vi "Camera.v6.vi"() -> ()   [LabVIEW 2015]
uses:
  Camera Properties.ctl
  Microscope Settings.ctl
  CameraState.ctl
  ModeEnum.ctl
  Stack_State.ctl
  Stack Track.ctl
  CameraControlTypeDef.ctl
  <vilib>/DAQmx/write.llb/DAQmx Write (Digital 1D Wfm NChan NSamp).vi
  <vilib>/DAQmx/write.llb/DAQmx Write (Analog 1D Wfm NChan NSamp).vi
  <vilib>/DAQmx/create/channels.llb/DAQmx Create Channel (AO-Voltage-Basic).vi
  <vilib>/Waveform/WDTOps.llb/WDT Number of Waveform Samples DBL.vi
  <vilib>/DAQmx/configure/timing.llb/DAQmx Timing (Sample Clock).vi
  <vilib>/Waveform/DWDTOps.llb/DWDT Uncompress Digital.vi
  <vilib>/DAQmx/miscellaneous.llb/DAQmx Fill In Error Info.vi
  <vilib>/vision/NI_Vision_Development_Module.lvlib
panel:
  in  "Tab Control":enum32{"Camera Settings", "Recording"}(tab)
  in  "Microscope Settings":T1={"Mode"=enum."XY", {"Scanning Mode"=12.0, "Slit Width /%"=5.0}, "Piezo Position /um"=0.0, "Exposure/ms"=40.0, "Samples per millisecond"=100.0, "Relax/ms"=10.0, "Readout Direction"=2.0, "Trigger Source"=2.0} {"Trigger Source" items=["Internal"=1.0, "External"=2.0]; "Readout Direction" items=["Forward"=1.0, "Backward"=2.0]; "?"."Scanning Mode" items=["Full Frame"=1.0, "Slit Scanning"=12.0]}
  in  "Scan":bool
  in  "Scan Continuously":bool
  out "error IO":errorcluster
  in  "V Height":dbl=2048.0 min=4.0 max=2048.0 step=4.0
  in  "V Offset":dbl min=0.0 max=0.0 step=4.0
  in  "H Offset":dbl min=0.0 max=0.0 step=4.0
  in  "H Width":dbl min=4.0 max=2048.0 step=4.0
  in  "Advanced DCAM Controls":i32(listbox) caption="Multicolumn Listbox"
  in  "Properties":T2=4211904 items=["SENSOR MODE"=4212128, "CCD MODE"=4212384, "READOUT MODE"=4211872, "ACTIVE VIEW INDEX"=4343136, "BITS PER CHANNEL"=4342976, "IMAGE PIXEL TYPE"=4343296, "BINNING"=4215968, "EXPOSURE TIME"=2049184, "CONTRAST GAIN"=3163312, "CONTRAST OFFSET"=3163328, "LIGHT MODE"=2114720, "SENSITIVITY"=2114992, "PHOTON IMAGING MODE"=2115200, "HIGH DYNAMIC RANGE MODE"=3163360, "WHITE BALANCE"=3163568, "TEMPERATURE"=2115232, "TEMPERATURE TARGET"=2115264, "SENSOR COOLER FAN"=2115296, "LINEBUNDLE HEIGHT"=4212192, "MECHANICAL SHUTTER"=2115488, "BACK FOCUS POSITION"=8422304, "TRIGGER CONNECTOR"=1066432, "TRIGGER SOURCE"=1066144, "OUTPUT TRIGGER SOURCE"=1852576, "TRIGGER GLOBAL EXPOSURE"=2049680, "FIRST TRIGGER BEHAVIOR"=2049696, "CHANNEL SYNC"=1852352, "READOUT DIRECTION"=4211904, "PRE HSYNC COUNT"=1852704, "INTERNAL LINE SPEED"=4191408, "INTERNAL LINE INVERVAL"=4191424]
  out "Waves":waveform(dbl)[](graph)
  out "Image":T3(plugin-control)
  out "Histogram":T4(graph)
  in  "stop":bool
  in  "Calibration":bool
  in  "MultiD Scan":bool
  in  "Stage Controller":bool
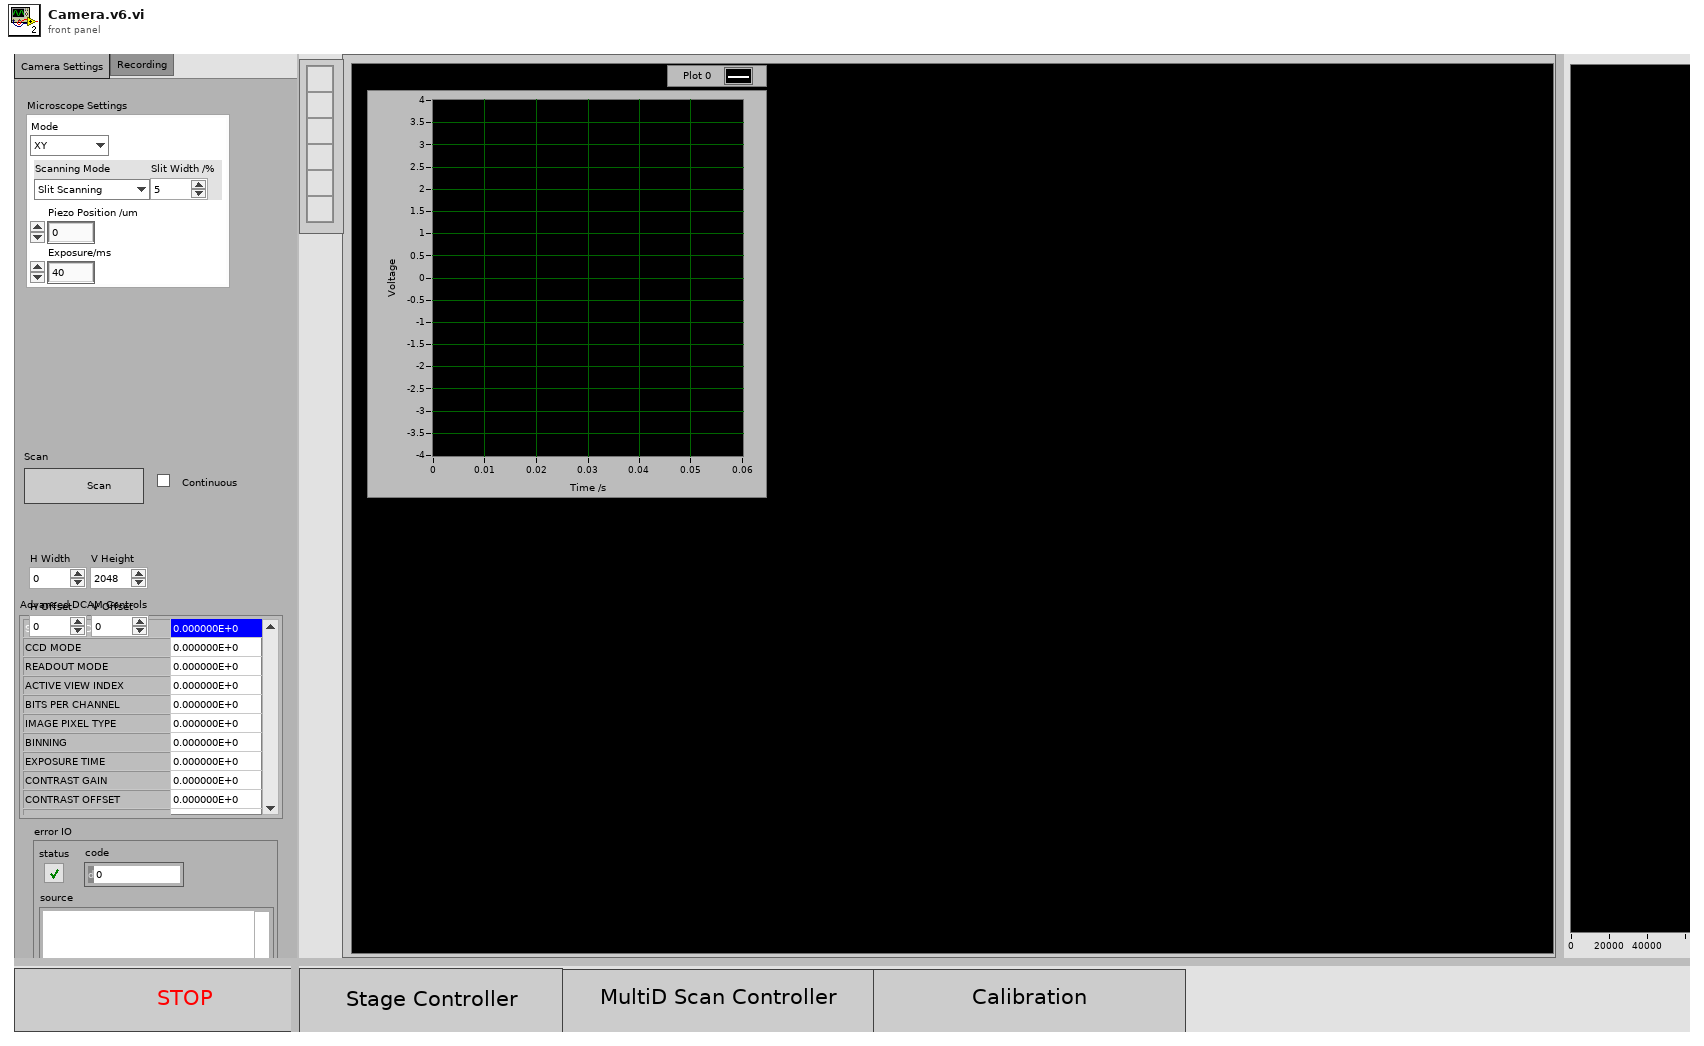
[diagram p1: front panel]
types:
  T1 = typedef "Microscope Settings.ctl" = cluster{"Mode":enum16{"X", "XY", "XYZ", "XYZT", "XYZC"}, cluster{"Scanning Mode":dbl, "Slit Width /%":dbl}, "Piezo Position /um":dbl, "Exposure/ms":dbl, "Samples per millisecond":dbl, "Relax/ms":dbl, "Readout Direction":dbl, "Trigger Source":dbl}
  T2 = typedef "Camera Properties.ctl" = u32
  T3 = typedef "IMAQ Image.ctl" = refnum<image>
  T4 = cluster{"Starting Value":sgl, "Incremental Value":sgl, "Histogram":u32[]}
  T5 = cluster{"height":u32, "width":u32, "datatype":u32}
  T6 = typedef "CameraState.ctl" = enum16{"init", "active", "deinit"}
  T7 = typedef "ModeEnum.ctl" = enum16{"Idle", "generateWaves", "runWaves", "stop"}
  T8 = typedef "CameraControlTypeDef.ctl" = enum16{"IntervalLineInt", "Ram Record", "HardDisk Record", "Disengage Update", "Update", "Idle", "ROI", "Binning", "Scan Mode", "Trigger Mode", "Readout Mode", "Readout Direction", "Preview", "ROIWindow", "Trigger Source"}
  T9 = typedef "Stack_State.ctl" = cluster{"State":T10, "Stack Number":i32, "Image":u16[][], "Stacks":i32}
  T10 = typedef "Stack Track.ctl" = enum16{"Idle", "Display", "Start Sequence", "Read Disk", "STOP", "Collecting", "End"}
  T11 = typedef "Image Type" = u32
  T12 = cluster{"Value":i32, "Minimum":i32, "Maximum":i32, "Increment":i32}
  T13 = cluster{"Minimum":i32, "Maximum":i32, "Increment":i32}
  T14 = cluster{"State":T10, "Timeout":i32, "Data 16":u16[][], "Timeout":i32}
  T15 = cluster{"Enum":T8, "Trigger Source":dbl, "timeout in ms (-1)":i32}
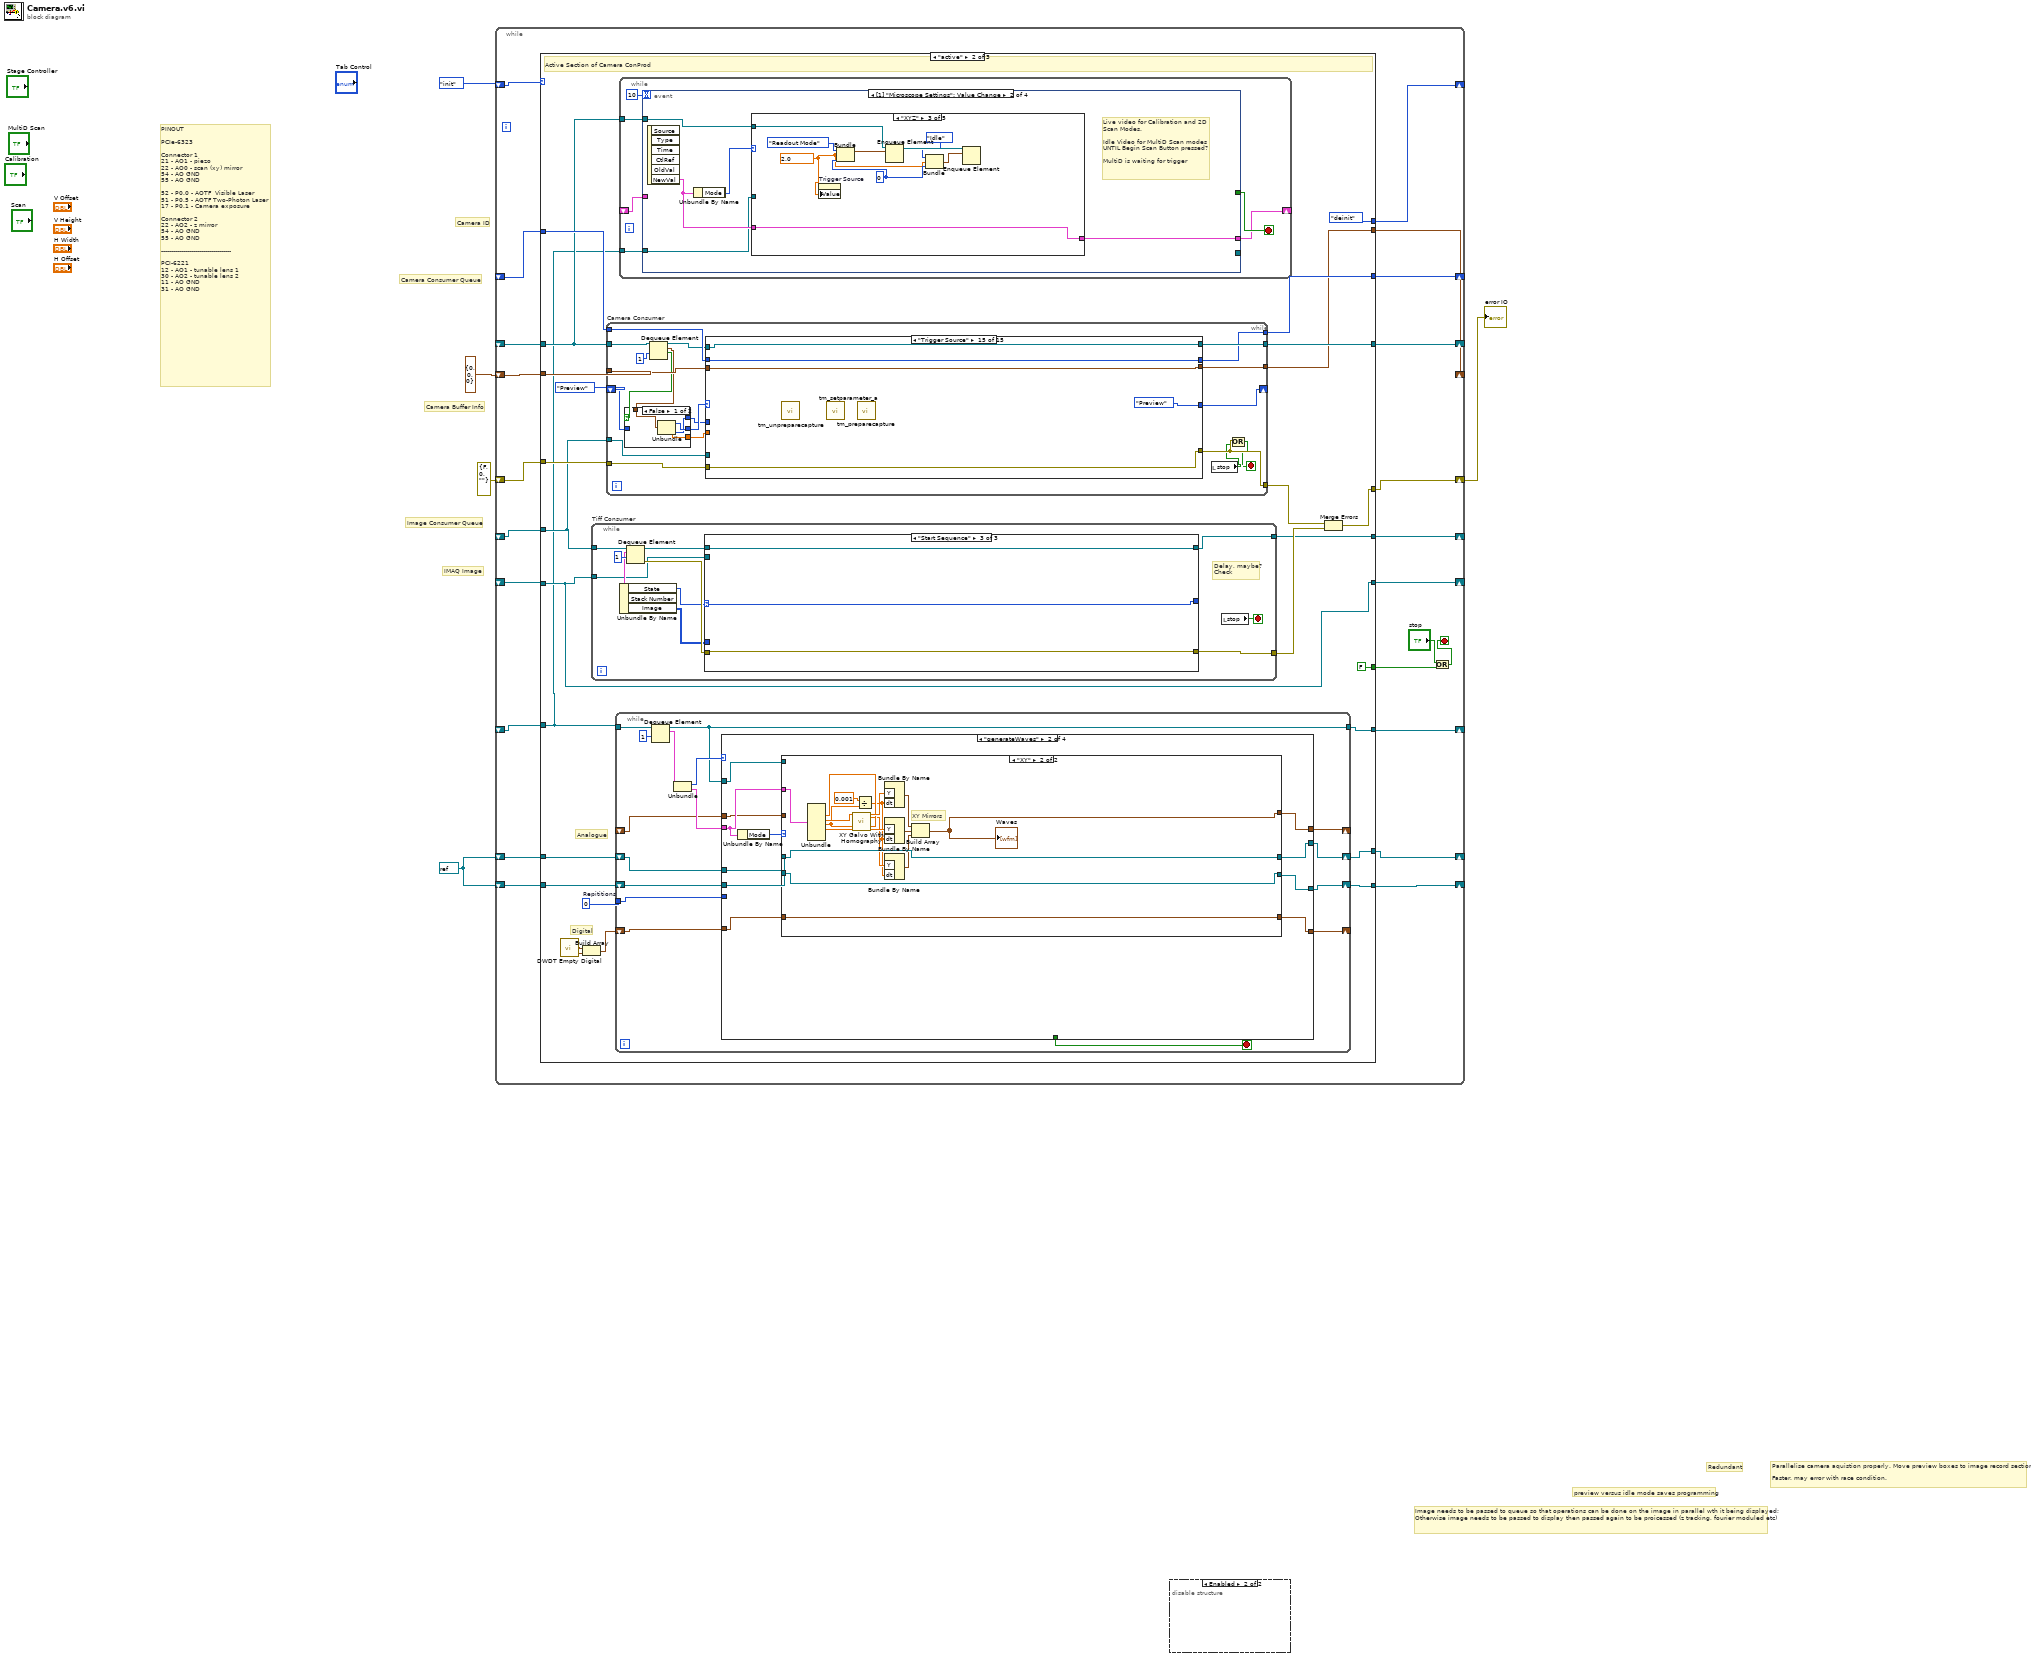
[diagram p0: block diagram]
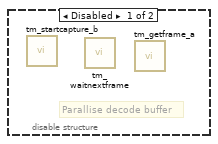
[diagram p2: hidden frame]
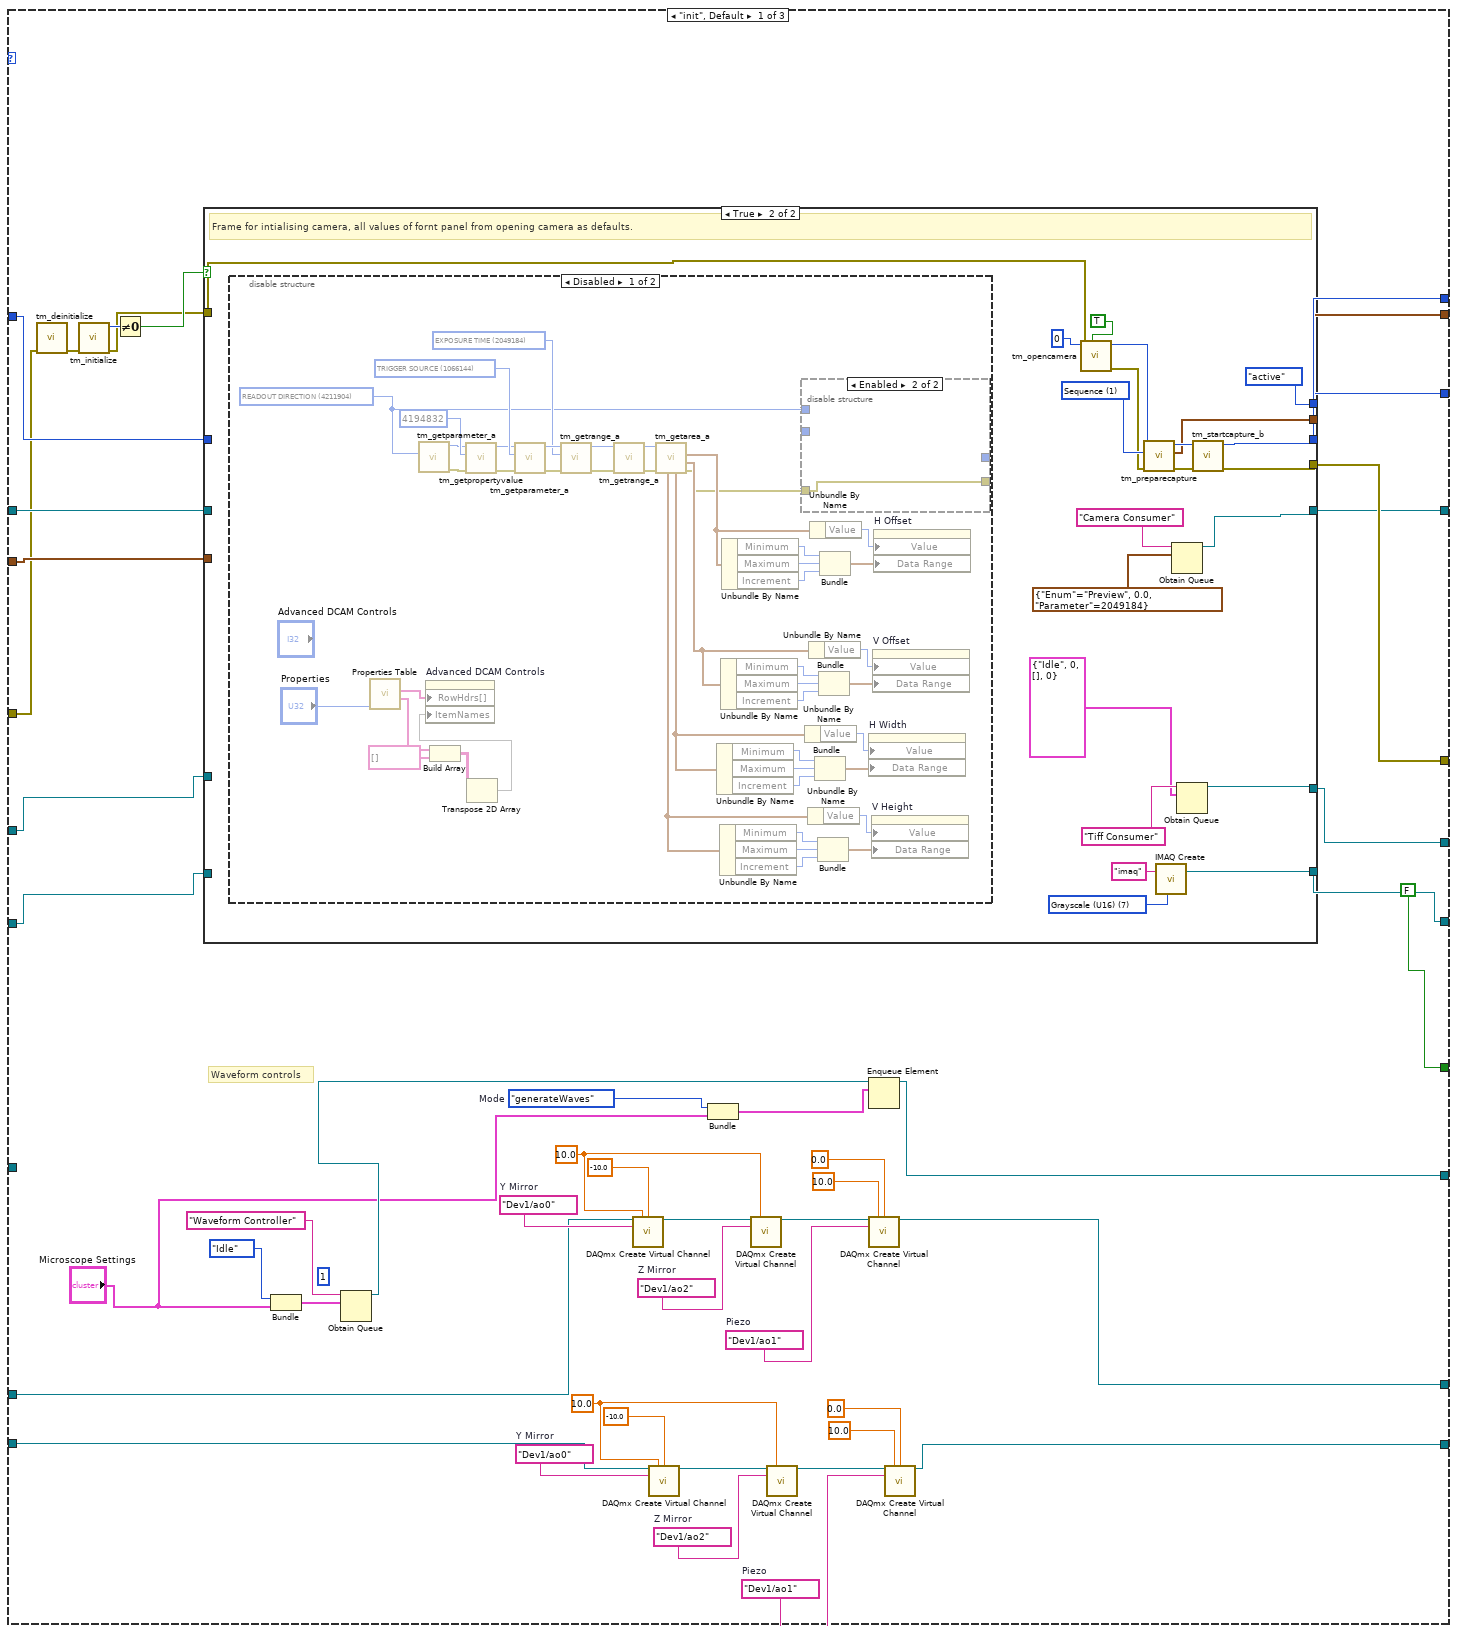
[diagram p3: hidden frame]
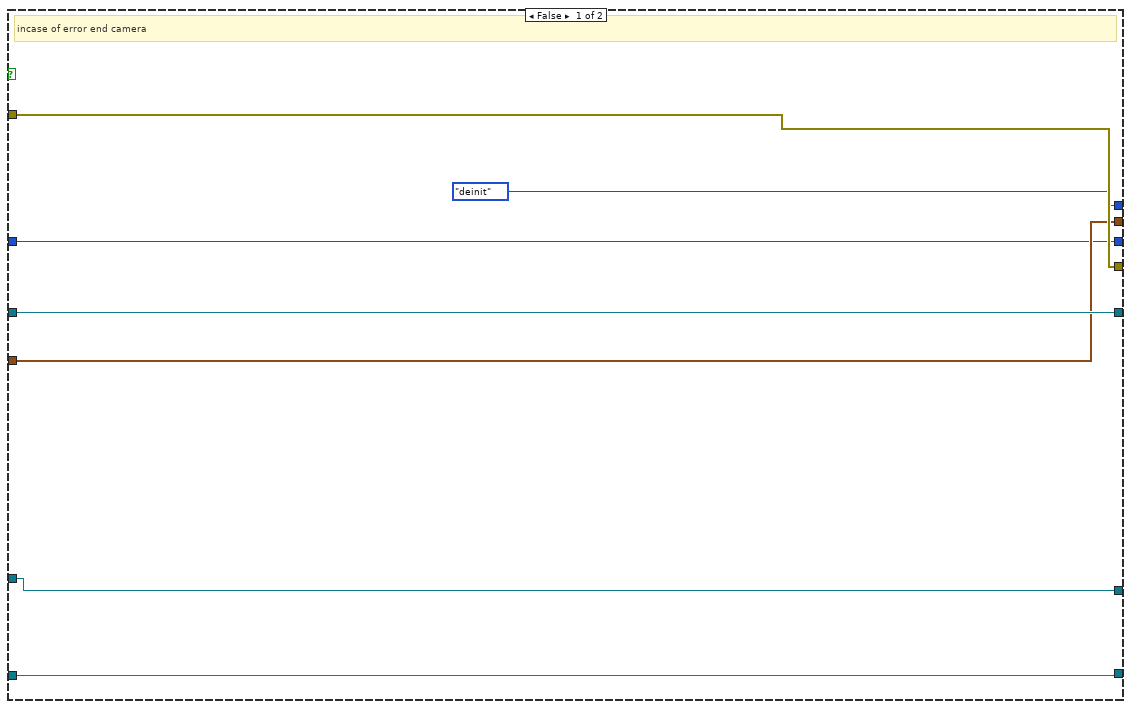
[diagram p4: hidden frame]
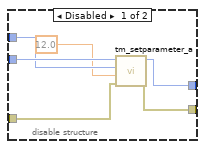
[diagram p5: hidden frame]
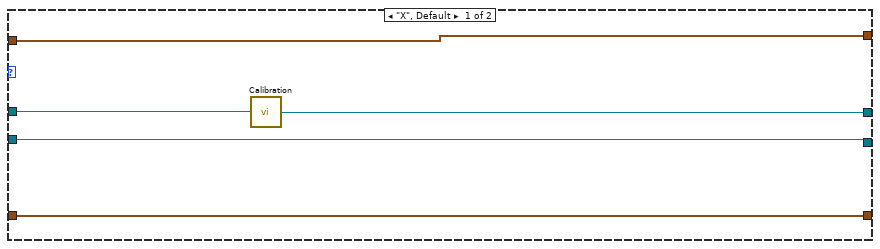
[diagram p8: hidden frame]
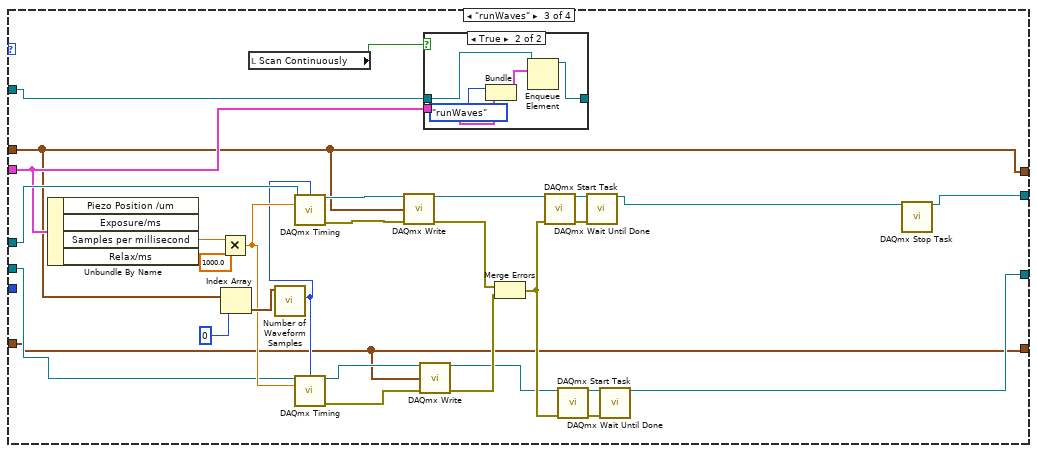
[diagram p9: hidden frame]
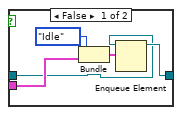
[diagram p10: hidden frame]
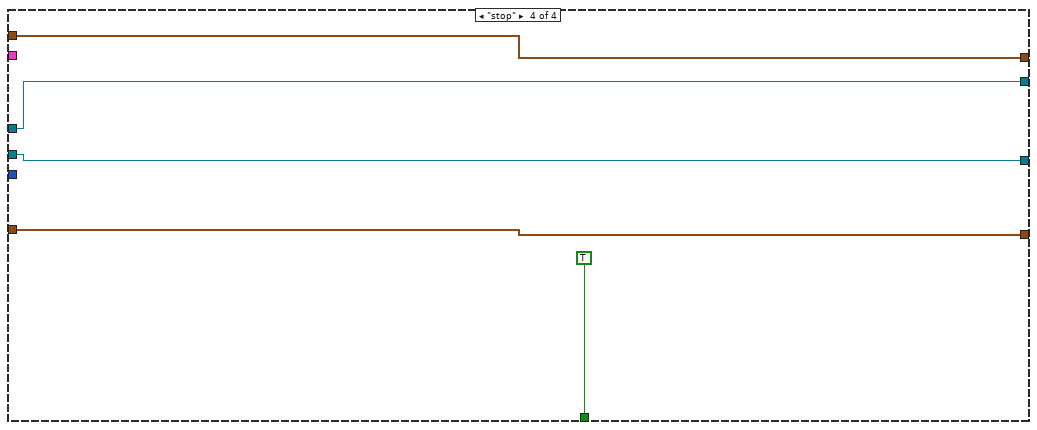
[diagram p11: hidden frame]
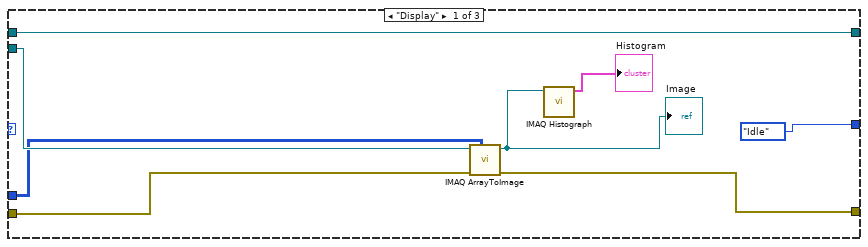
[diagram p12: hidden frame]
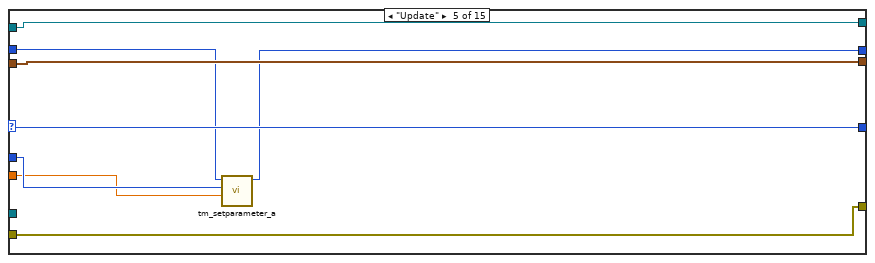
[diagram p19: hidden frame]
diagram:
  w2 = refnum<k21> refnum ("Mirror Z 2")
  # "PINOUT\n\nPCIe-6323\n\nConnector 1\n21 - AO1 - piezo\n22 - AO0 - scan (xy) mirror\n54 - AO GND\n55 - AO GND\n\n52 - P0.0 - AOTF  Visible Laser\n51 - P0.5 - AOTF Two-Photon Laser\n17 - P0.1 - Camera exposure\n\nConnector 2\n22 - AO2 - z mirror\n54 - AO GND\n55 - AO GND\n\n-----------------------------------\n\nPCI-6221\n12 - AO1 - tunable lens 1\n30 - AO2 - tunable lens 2\n11 - AO GND\n31 - AO GND"
  # "IMAQ Image"
  # "Camera Buffer Info"
  # "Image needs to be passed to queue so that operations can be done on the image in parallel wth it being displayed;\nOtherwise image needs to be passed to display then passed again to be proicessed (z tracking, fourier moduled etc)"
  # "preview versus idle mode saves programming"
  # "Parallelise camera aquistion properly. Move preview boxes to image record section.\n\nFaster. may error with race condition."
  # "Redundant"
  # "Image Consumer Queue"
  # "Camera Consumer Queue"
  # "Camera ID"
  n1 = while {
    shift-right: [w28] -> _
    shift-left: CameraState."init" -> [w27]
    shift-right: [w26] -> _
    shift-left: _ -> [w25]
    shift-right: [w24] -> w4
    shift-left: errorcluster {"status"=FALSE, "code"=0, "source"=""} ("error IO") -> [w23]
    shift-right: [w21] -> _
    shift-left: _ -> [w20]
    shift-right: [w22] -> _
    shift-left: _ -> [w19]
    shift-right: [w15] -> _
    shift-left: T5 {"height"=0, "width"=0, "datatype"=0} ("Buffer Info") -> [w14]
    shift-right: [w13] -> _
    shift-left: _ -> [w12]
    shift-right: [w11] -> _
    shift-left: w2 -> [w10]
    shift-right: [w8] -> _
    shift-left: w2 -> [w9]
    shift-right: [w7] -> _
    shift-left: _ -> [w6]
    stop <- w17 stop-if-true
    n2 = case shown="\"active\"" w27 {
      tunnel: [w72 CameraState."deinit" CameraState."init"] -> w28
      tunnel: [w71 w180 w490] -> w26
      tunnel: w25 -> [w49 w181 w490]
      tunnel: [w70 w179 w493] -> w24
      tunnel: w23 -> [w48 w173 w494]
      tunnel: [w69 w176 w477] -> w22
      tunnel: [w68 w175 w473] -> w21
      tunnel: w20 -> [w66 w168 w473]
      tunnel: w19 -> [w67 w166 w477]
      tunnel: [FALSE ("stop") FALSE ("stop") TRUE ("stop")] -> w16
      tunnel: [w64 w171 w487] -> w15
      tunnel: w14 -> [w63 w170 w487]
      tunnel: w12 -> [w61 w167 w486]
      tunnel: [w62 w167 w486] -> w13
      tunnel: w6 -> [_ w158 w472]
      tunnel: [w53 w159 w484] -> w11
      tunnel: w10 -> [w50 w162 w484]
      tunnel: w9 -> [w38 w161 w482]
      tunnel: [w37 w160 w482] -> w8
      tunnel: [w36 w157 w472] -> w7
      frame "init", Default {
        (unwired) 1 ("max queue size (-1, unlimited)")
        w34 = ModeEnum."generateWaves"  # Mode
        w43 = tag "Dev1/ao1"  # Piezo
        w44 = tag "Dev1/ao2"  # Z Mirror
        w45 = tag "Dev1/ao0"  # Y Mirror
        w47 = 10.0 ("maximum value")
        w56 = tag "Dev1/ao1"  # Piezo
        w57 = tag "Dev1/ao2"  # Z Mirror
        w58 = tag "Dev1/ao0"  # Y Mirror
        w60 = 10.0 ("maximum value")
        # "Waveform controls"
        n3 = call "tm_deinitialize.vi"("error in (no error)"=w48) -> ("error out"=w76:errorcluster)  [unwired: 10 in]
        n4 = call "tm_initialize.vi"("error in (no error)"=w76) -> ("error out"=w73:errorcluster, "Number Of Cameras"=w75:u32)  [unwired: 7 in, 2 out]
        n5 = Not Equal To 0?(x=w75) -> (x != 0?=w74:bool)
        n6 = case shown="True" w74 {
          tunnel: w73 -> [w83 w102]
          tunnel: [CameraState."deinit" CameraState."active"] -> w72
          tunnel: [w83 w99] -> w70
          tunnel: [w78 w97] -> w71
          tunnel: [w81 w84] -> w69
          tunnel: [w80 w94] -> w68
          tunnel: w67 -> [w81 _]
          tunnel: w66 -> [w80 _]
          tunnel: [w79 w92] -> w64
          tunnel: w63 -> [w79 _]
          tunnel: w49 -> [w78 _]
          tunnel: [w77 w89] -> w62
          tunnel: w61 -> [w77 _]
          frame False {
            # "incase of error end camera"
          }
          frame True {
            w91 = T11 7 items=["Grayscale (U8)", "Grayscale (I16)", "Grayscale (SGL)", "Complex (CSG)", "RGB (U32)", "HSL (U32)", "RGB (U64)", "Grayscale (U16)"] ("Image Type")
            w101 = 1 items=["Snap", "Sequence"] ("Capture mode")
            # "Frame for intialising camera, all values of fornt panel from opening camera as defaults."
            n7 = disable-structure shown="Disabled" {
              frame Disabled {
                w146 = u32 2049184 items=["SENSOR MODE"=4212128, "CCD MODE"=4212384, "READOUT MODE"=4211872, "ACTIVE VIEW INDEX"=4343136, "BITS PER CHANNEL"=4342976, "IMAGE PIXEL TYPE"=4343296, "BINNING"=4215968, "EXPOSURE TIME"=2049184, "CONTRAST GAIN"=3163312, "CONTRAST OFFSET"=3163328, "LIGHT MODE"=2114720, "SENSITIVITY"=2114992, "PHOTON IMAGING MODE"=2115200, "HIGH DYNAMIC RANGE MODE"=3163360, "WHITE BALANCE"=3163568, "TEMPERATURE"=2115232, "TEMPERATURE TARGET"=2115264, "SENSOR COOLER FAN"=2115296, "LINEBUNDLE HEIGHT"=4212192, "MECHANICAL SHUTTER"=2115488, "BACK FOCUS POSITION"=8422304, "TRIGGER CONNECTOR"=1066432, "TRIGGER SOURCE"=1066144, "OUTPUT TRIGGER SOURCE"=1852576, "TRIGGER GLOBAL EXPOSURE"=2049680, "FIRST TRIGGER BEHAVIOR"=2049696, "CHANNEL SYNC"=1852352, "READOUT DIRECTION"=4211904, "PRE HSYNC COUNT"=1852704, "INTERNAL LINE SPEED"=4191408, "INTERNAL LINE INVERVAL"=4191424] ("Parameter")
                w106 = T2 4211904 items=["SENSOR MODE"=4212128, "CCD MODE"=4212384, "READOUT MODE"=4211872, "ACTIVE VIEW INDEX"=4343136, "BITS PER CHANNEL"=4342976, "IMAGE PIXEL TYPE"=4343296, "BINNING"=4215968, "EXPOSURE TIME"=2049184, "CONTRAST GAIN"=3163312, "CONTRAST OFFSET"=3163328, "LIGHT MODE"=2114720, "SENSITIVITY"=2114992, "PHOTON IMAGING MODE"=2115200, "HIGH DYNAMIC RANGE MODE"=3163360, "WHITE BALANCE"=3163568, "TEMPERATURE"=2115232, "TEMPERATURE TARGET"=2115264, "SENSOR COOLER FAN"=2115296, "LINEBUNDLE HEIGHT"=4212192, "MECHANICAL SHUTTER"=2115488, "BACK FOCUS POSITION"=8422304, "TRIGGER CONNECTOR"=1066432, "TRIGGER SOURCE"=1066144, "OUTPUT TRIGGER SOURCE"=1852576, "TRIGGER GLOBAL EXPOSURE"=2049680, "FIRST TRIGGER BEHAVIOR"=2049696, "CHANNEL SYNC"=1852352, "READOUT DIRECTION"=4211904, "PRE HSYNC COUNT"=1852704, "INTERNAL LINE SPEED"=4191408, "INTERNAL LINE INVERVAL"=4191424] ("Parameter")
                w149 = u32 1066144 items=["SENSOR MODE"=4212128, "CCD MODE"=4212384, "READOUT MODE"=4211872, "ACTIVE VIEW INDEX"=4343136, "BITS PER CHANNEL"=4342976, "IMAGE PIXEL TYPE"=4343296, "BINNING"=4215968, "EXPOSURE TIME"=2049184, "CONTRAST GAIN"=3163312, "CONTRAST OFFSET"=3163328, "LIGHT MODE"=2114720, "SENSITIVITY"=2114992, "PHOTON IMAGING MODE"=2115200, "HIGH DYNAMIC RANGE MODE"=3163360, "WHITE BALANCE"=3163568, "TEMPERATURE"=2115232, "TEMPERATURE TARGET"=2115264, "SENSOR COOLER FAN"=2115296, "LINEBUNDLE HEIGHT"=4212192, "MECHANICAL SHUTTER"=2115488, "BACK FOCUS POSITION"=8422304, "TRIGGER CONNECTOR"=1066432, "TRIGGER SOURCE"=1066144, "OUTPUT TRIGGER SOURCE"=1852576, "TRIGGER GLOBAL EXPOSURE"=2049680, "FIRST TRIGGER BEHAVIOR"=2049696, "CHANNEL SYNC"=1852352, "READOUT DIRECTION"=4211904, "PRE HSYNC COUNT"=1852704, "INTERNAL LINE SPEED"=4191408, "INTERNAL LINE INVERVAL"=4191424] ("Parameter")
                n8 = call "Properties Table.vi"("Properties"="Properties") -> ("Value Stirngs Out"=w111:string[], "Row Headers"=w112:string[])  [unwired: 4 in, 2 out]
                n9 = call "tm_getparameter_a.vi"("Parameter"=w106) -> ("error out"=w138:errorcluster, "Handle out"=w140:u32)  [unwired: 8 in, 1 out]
                n10 = Build Array(w111, string[] [] ("element")) -> (w109:string[][])
                n11 = call "tm_getpropertyvalue.vi"("error in (no error)"=w138, "Property ID"=u32 4194832, "Handle in"=w140) -> ("error out"=w139:errorcluster, "Handle out"=w105:u32)  [unwired: 6 in, 1 out]
                n12 = Transpose 2D Array(2D array=w109) -> (transposed array=w108:string[][])
                n13 = property on="Advanced DCAM Controls" class="MCListbox (strict)"("RowHdrs[]"=w112, "ItemNames"=w108) -> ()  [unwired: 2 in, 2 out]
                n14 = call "tm_getparameter_a.vi"("error in (no error)"=w139, "Parameter"=w149, "Handle in"=w105) -> ("error out"=w147:errorcluster, "Handle out"=w148:u32)  [unwired: 6 in, 1 out]
                n15 = call "tm_getrange_a.vi"("error in (no error)"=w147, "Parameter"=w146, "Handle in"=w148) -> ("error out"=w144:errorcluster, "Handle out"=w145:u32)  [unwired: 2 in, 5 out]
                n16 = call "tm_getrange_a.vi"("error in (no error)"=w144, "Handle in"=w145) -> ("error out"=w143:errorcluster, "Handle out"=w142:u32)  [unwired: 3 in, 5 out]
                n17 = call "tm_getarea_a.vi"("error in (no error)"=w143, "Handle in"=w142) -> ("error out"=w107:errorcluster, "V Offset"=w114:T12, "H Offset"=w137:T12, "H Width"=w115:T12, "V Width"=w116:T12)  [unwired: 4 in, 1 out]
                n18 = Unbundle By Name(w115) -> ("Minimum"=w126:i32, "Maximum"=w125:i32, "Increment"=w124:i32)
                n19 = Unbundle By Name(w116) -> ("Minimum"=w117:i32, "Maximum"=w118:i32, "Increment"=w119:i32)
                n20 = Unbundle By Name(w114) -> ("Minimum"=w127:i32, "Maximum"=w128:i32, "Increment"=w129:i32)
                n21 = Unbundle By Name(w137) -> ("Minimum"=w136:i32, "Maximum"=w135:i32, "Increment"=w134:i32)
                n22 = disable-structure shown="Enabled" {
                  disable-tunnel: _ -> [w155 _]
                  disable-tunnel: [w154 _] -> _
                  disable-tunnel: w107 -> [w153 w156]
                  disable-tunnel: [w152 w156] -> _
                  disable-tunnel: w106 -> [w151 _]
                  frame Disabled {
                    n23 = call "tm_setparameter_a.vi"("error in (no error)"=w153, "Value in"=12.0, "Parameter"=w151, "Handle in"=w155) -> ("error out"=w152:errorcluster, "Handle out"=w154:u32)  [unwired: 6 in]
                  }
                  frame Enabled {
                  }
                }
                n24 = Unbundle By Name(w115) -> ("Value"=w122:i32)
                n25 = Unbundle By Name(w116) -> ("Value"=w121:i32)
                n26 = Unbundle By Name(w114) -> ("Value"=w131:i32)
                n27 = Unbundle By Name(w137) -> ("Value"=w132:i32)
                n28 = Bundle("Minimum"=w126, "Maximum"=w125, "Increment"=w124) -> (w123:T13)  [unwired: 1 in]
                n29 = Bundle("Minimum"=w117, "Maximum"=w118, "Increment"=w119) -> (w120:T13)  [unwired: 1 in]
                n30 = Bundle("Minimum"=w127, "Maximum"=w128, "Increment"=w129) -> (w130:T13)  [unwired: 1 in]
                n31 = Bundle("Minimum"=w136, "Maximum"=w135, "Increment"=w134) -> (w133:T13)  [unwired: 1 in]
                n32 = property on="H Width" class="DigNum (strict)"("Value"=w122, "Data Range"=w123) -> ()  [unwired: 2 in, 2 out]
                n33 = property on="V Height" class="DigNum (strict)"("Value"=w121, "Data Range"=w120) -> ()  [unwired: 2 in, 2 out]
                n34 = property on="V Offset" class="DigNum (strict)"("Value"=w131, "Data Range"=w130) -> ()  [unwired: 2 in, 2 out]
                n35 = property on="H Offset" class="DigNum (strict)"("Value"=w132, "Data Range"=w133) -> ()  [unwired: 2 in, 2 out]
              }
              frame Enabled {
              }
            }
            n36 = call "tm_opencamera.vi"("Force Open"=TRUE, "error in (no error)"=w102, "Camera Index"=u32 0) -> ("error out"=w86:errorcluster, "Handle out"=w85:u32)  [unwired: 6 in, 1 out]
            n37 = call "tm_preparecapture.vi"("error in (no error)"=w86, "Capture mode"=w101, "Handle in"=w85) -> ("error out"=w100:errorcluster, "Buffer Info"=w92:T5, "Handle out"=w98:u32)  [unwired: 5 in, 1 out]
            n38 = call "IMAQ Create"("Image Name"="imaq", "Image Type"=w91) -> ("New Image"=w89:T3)  [unwired: 3 in, 1 out]
            n39 = Obtain Queue(name (unnamed)="Camera Consumer", element data type=cluster{"Enum":T8, dbl, "Parameter":u32} {"Enum"=enum."Preview", 0.0, "Parameter"=2049184}) -> (queue out=w84:refnum<queue>)  [unwired: 3 in, 2 out]
            n40 = Obtain Queue(name (unnamed)="Tiff Consumer", element data type=T9 {"State"=enum."Idle", "Stack Number"=0, "Image"=[], "Stacks"=0} ("input cluster")) -> (queue out=w94:refnum<queue>)  [unwired: 3 in, 2 out]
            n41 = call "tm_startcapture_b.vi"("error in (no error)"=w100, "Handle in"=w98) -> ("error out"=w99:errorcluster, "Handle out"=w97:u32)  [unwired: 8 in]
          }
        }
        n42 = Bundle("Mode"=ModeEnum."Idle", "Microscope Settings"="Microscope Settings") -> (w31:cluster{"Mode":T7, "Microscope Settings":T1})  [unwired: 1 in]
        n43 = Obtain Queue(name (unnamed)="Waveform Controller", element data type=w31) -> (queue out=w30:refnum<queue>)  [unwired: 3 in, 2 out]
        n44 = call-poly <vilib>:"DAQmx Create Virtual Channel.vi"("task in"=w50, "maximum value"=w60, "minimum value"=-10.0, "physical channels"=w58) -> ("task out"=w52:refnum<k21>)  [unwired: 10 in, 1 out]
        n45 = call-poly <vilib>:"DAQmx Create Virtual Channel.vi"("task in"=w38, "maximum value"=w47, "minimum value"=-10.0, "physical channels"=w45) -> ("task out"=w40:refnum<k21>)  [unwired: 10 in, 1 out]
        n46 = Bundle("Mode"=w34, "Microscope Settings"="Microscope Settings") -> (w35:cluster{"Mode":T7, "Microscope Settings":T1})  [unwired: 1 in]
        n47 = call-poly <vilib>:"DAQmx Create Virtual Channel.vi"("task in"=w52, "maximum value"=w60, "physical channels"=w57) -> ("task out"=w51:refnum<k21>)  [unwired: 11 in, 1 out]
        n48 = call-poly <vilib>:"DAQmx Create Virtual Channel.vi"("task in"=w40, "maximum value"=w47, "physical channels"=w44) -> ("task out"=w39:refnum<k21>)  [unwired: 11 in, 1 out]
        n49 = Enqueue Element(queue=w30, element=w35) -> (queue out=w36:refnum<queue>)  [unwired: 2 in, 2 out]
        n50 = call-poly <vilib>:"DAQmx Create Virtual Channel.vi"("task in"=w51, "maximum value"=10.0 ("minimum value"), "minimum value"=0.0 ("maximum value"), "physical channels"=w56) -> ("task out"=w53:refnum<k21>)  [unwired: 10 in, 1 out]
        n51 = call-poly <vilib>:"DAQmx Create Virtual Channel.vi"("task in"=w39, "maximum value"=10.0 ("minimum value"), "minimum value"=0.0 ("maximum value"), "physical channels"=w43) -> ("task out"=w37:refnum<k21>)  [unwired: 10 in, 1 out]
      }
      frame "active" {
        w165 = 0  # Repititions
        # "Digital"
        # "Analogue"
        # "Active Section of Camera ConProd"
        n52 = call <vilib>:"DWDT Empty Digital.vi"() -> ("digital waveform out"=w163:digitalwaveform)  [unwired: 5 in]
        n53 = Build Array(w163, w163) -> (w164:digitalwaveform[])
        n54 = while "Tiff Consumer" {
          tunnel: [w282] -> w178
          tunnel: [w285] -> w175
          tunnel: w168 -> [w287]
          tunnel: w167 -> [w279]
          stop <- w289 stop-if-true
          # "Delay, maybe?\nCheck"
          n55 = Dequeue Element(queue=w287, timeout in ms (-1)=1) -> (queue out=w284:refnum<queue>, element=w286:T9, error out=w283:errorcluster)  [unwired: 1 in, 1 out]
          n56 = Unbundle By Name(w286) -> ("State"=w280:T10, "Image"=w281:u16[][])  [unwired: 1 out]
          n57 = case shown="\"Start Sequence\"" w280 {
            selector: w280 -> [_ w300 w301]
            tunnel: [w297 w299 w302] -> w285
            tunnel: w284 -> [w297 w299 w302]
            tunnel: [Stack_Track."Idle" ("State") w300 w301] -> _
            tunnel: w281 -> [w292 _ _]
            tunnel: w279 -> [w296 _ _]
            tunnel: w283 -> [w295 w298 w303]
            tunnel: [w294 w298 w303] -> w282
            frame "Display" {
              n58 = call "IMAQ ArrayToImage"("Image Pixels (U16)"=w292, "error in (no error)"=w295, "Image"=w296) -> ("error out"=w294:errorcluster, "Image Out"=w291:T3)  [unwired: 7 in]
              "Image" <- w291
              n59 = call "IMAQ Histograph"("Image"=w291) -> ("Histogram Graph"=→"Histogram":T4)  [unwired: 7 in, 3 out]
            }
            frame "Idle", Default {
            }
            frame "Start Sequence" {
            }
          }
          n60 = local read "stop"() -> (w289:bool)
        }
        n61 = while "Camera Consumer" {
          tunnel: w173 -> [w322]
          tunnel: w181 -> [w320]
          tunnel: [w319] -> w180
          tunnel: [w306] -> w177
          tunnel: w166 -> [w315]
          tunnel: [w323] -> w176
          shift-right: [w321] -> _
          shift-left: CameraControlTypeDef."Preview" ("Enum") -> [w311]
          tunnel: [w318] -> w171
          tunnel: w170 -> [w317]
          tunnel: w168 -> [w310]
          stop <- w304 stop-if-true
          n62 = Dequeue Element(queue=w315, timeout in ms (-1)=1) -> (queue out=w314:refnum<queue>, element=w309:cluster{"Enum":T8, dbl, "Parameter":u32}, timed out?=w313:bool)  [unwired: 1 in, 1 out]
          n63 = case shown="False" w313 {
            tunnel: [w326 w328] -> w312
            tunnel: w311 -> [_ w328]
            tunnel: w309 -> [w327 _]
            tunnel: [w325 _] -> w308
            tunnel: [w324 w328] -> w307
            frame False {
              n64 = Unbundle(w327) -> ("Enum"=w326:T8, w325:dbl, "Parameter"=w324:u32)
            }
            frame True {
            }
          }
          n65 = case shown="\"Trigger Source\"" w312 {
            selector: w312 -> [w332 w337 w342 w347 w355 w360 w365 w370 w375 w380 w385 w390 _ w411 _]
            tunnel: w314 -> [w331 w338 w343 w348 w356 w361 w366 w371 w376 w381 w386 w391 w408 w413 w418]
            tunnel: [w331 w338 w343 w348 w356 w361 w366 w371 w376 w381 w386 w391 w408 w413 w418] -> w323
            tunnel: w322 -> [w333 w336 w341 w346 w354 w359 w364 w369 w374 w379 w384 w389 w395 w410 w416]
            tunnel: [w333 w336 w341 w346 w354 w359 w364 w369 w374 w379 w384 w389 w392 w410 w416] -> w306
            tunnel: [w332 w337 w342 w347 w355 w360 w365 w370 w375 w380 w385 w390 CameraControlTypeDef."Preview" ("Enum") w411 CameraControlTypeDef."Preview" ("Enum")] -> w321
            tunnel: w320 -> [w330 w335 w340 w345 w352 w358 w363 w368 w373 w378 w383 w388 w406 w412 w417]
            tunnel: [w330 w335 w340 w345 w351 w358 w363 w368 w373 w378 w383 w388 w404 w412 w417] -> w319
            tunnel: [w329 w334 w339 w344 w353 w357 w362 w367 w372 w377 w382 w387 w401 w409 w415] -> w318
            tunnel: w317 -> [w329 w334 w339 w344 w353 w357 w362 w367 w372 w377 w382 w387 w401 w409 w415]
            tunnel: w310 -> [_ _ _ _ _ _ _ _ _ _ _ _ w400 _ _]
            tunnel: w308 -> [_ _ _ _ w349 _ _ _ _ _ _ _ _ _ _]
            tunnel: w307 -> [_ _ _ _ w350 _ _ _ _ _ _ _ _ _ _]
            frame "IntervalLineInt" {
            }
            frame "Ram Record" {
            }
            frame "HardDisk Record" {
            }
            frame "Disengage Update" {
            }
            frame "Update" {
              n66 = call "tm_setparameter_a.vi"("Value in"=w349, "Parameter"=w350, "Handle in"=w352) -> ("Handle out"=w351:u32)  [unwired: 7 in, 1 out]
            }
            frame "Idle", Default {
            }
            frame "ROI" {
            }
            frame "Binning" {
            }
            frame "Scan Mode" {
            }
            frame "Trigger Mode" {
            }
            frame "Readout Mode" {
            }
            frame "Readout Direction" {
            }
            frame "Preview" {
              w397 = 0 ("Timeout")
              n67 = call "tm_waitnextframe.vi"("error in (no error)"=w395, "Timeout"=3000, "Handle in"=w406) -> ("error out"=w403:errorcluster, "Handle out"=w405:u32)  [unwired: 5 in, 2 out]
              n68 = call "tm_getframe_a.vi"("error in (no error)"=w403, "Buffer Info"=w401, "Handle in"=w405) -> ("error out"=w393:errorcluster, "Data 16"=w398:u16[][], "Handle out"=w404:u32)  [unwired: 4 in, 2 out]
              n69 = Bundle("State"=Stack_Track."Display", "Timeout"=w397, "Data 16"=w398, "Timeout"=w397) -> (w396:T14)  [unwired: 1 in]
              n70 = Enqueue Element(queue=w400, element=w396, error in (no error)=w395) -> (error out=w394:errorcluster)  [unwired: 1 in, 2 out]
              n71 = Merge Errors(w393, w394) -> (w392:errorcluster)
            }
            frame "ROIWindow" {
            }
            frame "Trigger Source" {
              n72 = call "tm_unpreparecapture.vi"() -> ()  [unwired: 10 in, 2 out]
              n73 = call "tm_setparameter_a.vi"() -> ()  [unwired: 10 in, 2 out]
              n74 = call "tm_preparecapture.vi"() -> ()  [unwired: 8 in, 4 out]
            }
          }
          n75 = local read "stop"() -> (w305:bool)
          n76 = Or(x=w306, y=w305) -> (x .or. y?=w304:bool)
        }
        n77 = while {
          tunnel: w158 -> [w197]
          shift-right: [w192] -> _
          shift-left: _ -> [w191]
          tunnel: w165 -> [w190]
          shift-right: [w186] -> w159
          shift-left: w162 -> [w185]
          shift-right: [w189] -> _
          shift-left: w164 -> [w188]
          shift-right: [w184] -> w160
          shift-left: w161 -> [w183]
          tunnel: [w182] -> w157
          stop <- w196 stop-if-true
          n78 = Dequeue Element(queue=w197, timeout in ms (-1)=1) -> (queue out=w182:refnum<queue>, element=w195:cluster{"Mode":T7, "Microscope Settings":T1})  [unwired: 1 in, 2 out]
          n79 = Unbundle(w195) -> ("Mode"=w194:T7, "Microscope Settings"=w193:T1)
          n80 = case shown="\"generateWaves\"" w194 {
            tunnel: [_ _ _ TRUE] -> w196
            tunnel: w193 -> [_ w211 w258 _]
            tunnel: [w201 w212 w257 w278] -> w192
            tunnel: w191 -> [w201 w203 w257 w278]
            tunnel: w190 -> [_ _ _ _]
            tunnel: w182 -> [_ w202 w259 _]
            tunnel: [w198 w207 w243 w277] -> w184
            tunnel: [w199 w205 w252 w276] -> w186
            tunnel: w185 -> [w199 w204 w260 w276]
            tunnel: [w200 w210 w235 w275] -> w189
            tunnel: w188 -> [w200 w209 w235 w275]
            tunnel: w183 -> [w198 w208 w245 w277]
            frame "Idle", Default {
            }
            frame "generateWaves" {
              n81 = Unbundle By Name(w211) -> ("Mode"=w206:enum16{"X", "XY", "XYZ", "XYZT", "XYZC"})
              n82 = case shown="\"XY\"" w206 {
                tunnel: [w217 w221] -> w212
                tunnel: w211 -> [_ w224]
                tunnel: [w215 w227] -> w210
                tunnel: w209 -> [w215 w227]
                tunnel: w208 -> [w216 w226]
                tunnel: [w216 w226] -> w207
                tunnel: [w213 w225] -> w205
                tunnel: w204 -> [w214 w225]
                tunnel: w203 -> [w217 _]
                tunnel: w202 -> [_ _]
                frame "X", Default {
                  n83 = call "Calibration.vi"("Analogue In"=w214) -> ("Analogue In Out"=w213:refnum<k21>)
                }
                frame "XY" {
                  # "XY Mirrors"
                  n84 = Unbundle(w224) -> ("Piezo Position /um"=w230:dbl, "Exposure/ms"=w228:dbl, "Samples per millisecond"=w219:dbl, "Relax/ms"=w229:dbl)  [unwired: 4 out]
                  n85 = call "XY Galvo With Homography.vi"("Exposure (ms)"=w228, "Samples /Millisecond"=w219, "Relax (ms)"=w229, "Piezo Position (um)"=w230) -> ("Scan Mirror Signal"=w234:dbl[], "Piezo Signal"=w223:dbl[], "Z Mirror Signal"=w233:dbl[])  [unwired: 11 in, 2 out]
                  n86 = Divide(x=0.001 ("y"), y=w219) -> (x/y=w220:dbl)
                  n87 = Bundle By Name("Y"=w234, "dt"=w220) -> (w231:waveform(dbl))  [unwired: 1 in]
                  n88 = Bundle By Name("Y"=w233, "dt"=w220) -> (w232:waveform(dbl))  [unwired: 1 in]
                  n89 = Bundle By Name("Y"=w223, "dt"=w220) -> (w222:waveform(dbl))  [unwired: 1 in]
                  n90 = Build Array(w231, w232, w222) -> (w221:waveform(dbl)[])
                  "Waves" <- w221
                }
              }
            }
            frame "runWaves" {
              n91 = Unbundle By Name(w258) -> ("Samples per millisecond"=w251:dbl)  [unwired: 3 out]
              n92 = Multiply(x=w251, y=1000.0) -> (x*y=w248:dbl)
              n93 = Index Array(array=w257, index=0) -> (element=w255:waveform(dbl))
              n94 = local read "Scan Continuously"() -> (w249:bool)
              n95 = call-poly <vilib>:"Number of Waveform Samples.vi"("waveform in"=w255) -> ("number of samples"=w247:i32)  [unwired: 8 in, 2 out]
              n96 = call-poly <vilib>:"DAQmx Timing.vi"("task/channels in"=w260, "samples per channel"=w247, "rate"=w248) -> ("task out"=w263:refnum<k21>, "error out"=w254:errorcluster)  [unwired: 11 in]
              n97 = call-poly <vilib>:"DAQmx Timing.vi"("task/channels in"=w245, "samples per channel"=w247, "rate"=w248) -> ("task out"=w246:refnum<k21>, "error out"=w242:errorcluster)  [unwired: 11 in]
              n98 = call-poly <vilib>:"DAQmx Write.vi"("task/channels in"=w263, "data"=w257, "error in"=w254) -> ("task out"=w237:refnum<k21>, "error out"=w240:errorcluster)  [unwired: 10 in, 1 out]
              n99 = call-poly <vilib>:"DAQmx Write.vi"("task/channels in"=w246, "data"=w235, "error in"=w242) -> ("task out"=w236:refnum<k21>, "error out"=w239:errorcluster)  [unwired: 10 in, 1 out]
              n100 = case shown="True" w249 {
                tunnel: w259 -> [w265 w273]
                tunnel: [w266 w272] -> _
                tunnel: w258 -> [w267 w271]
                frame False {
                  n101 = Bundle("Mode"=ModeEnum."Idle", "Microscope Settings"=w267) -> (w268:cluster{"Mode":T7, "Microscope Settings":T1})  [unwired: 1 in]
                  n102 = Enqueue Element(queue=w265, element=w268) -> (queue out=w266:refnum<queue>)  [unwired: 2 in, 2 out]
                }
                frame True {
                  n103 = Bundle("Mode"=ModeEnum."runWaves", "Microscope Settings"=w271) -> (w270:cluster{"Mode":T7, "Microscope Settings":T1})  [unwired: 1 in]
                  n104 = Enqueue Element(queue=w273, element=w270) -> (queue out=w272:refnum<queue>)  [unwired: 2 in, 2 out]
                }
              }
              n105 = Merge Errors(w240, w239) -> (w238:errorcluster)
              n106 = call <vilib>:"DAQmx Start Task.vi"("task/channels in"=w237, "error in"=w238) -> ("task out"=w262:refnum<k21>, "error out"=w261:errorcluster)  [unwired: 12 in]
              n107 = call <vilib>:"DAQmx Start Task.vi"("task/channels in"=w236, "error in"=w238) -> ("task out"=w244:refnum<k21>, "error out"=w241:errorcluster)  [unwired: 12 in]
              n108 = call <vilib>:"DAQmx Wait Until Done.vi"("task/channels in"=w262, "error in"=w261) -> ("task out"=w253:refnum<k21>)  [unwired: 12 in, 1 out]
              n109 = call <vilib>:"DAQmx Wait Until Done.vi"("task/channels in"=w244, "error in"=w241) -> ("task out"=w243:refnum<k21>)  [unwired: 12 in, 1 out]
              n110 = call <vilib>:"DAQmx Stop Task.vi"("task/channels in"=w253) -> ("task out"=w252:refnum<k21>)  [unwired: 13 in, 1 out]
            }
            frame "stop" {
            }
          }
        }
        n111 = while {
          tunnel: w166 -> [w423]
          shift-right: [w422] -> _
          shift-left: _ -> [w421]
          tunnel: w158 -> [w419]
          stop <- w424 stop-if-true
          n112 = event shown="[1] \"Microscope Settings\": Value Change" {
            selector: _ -> [_ _ _ _]
            dyn-events: _ -> [_ _ _ _]
            timeout: 10 -> [_ _ _ _]
            tunnel: [w425 _ _ _] -> w424
            tunnel: w423 -> [_ w430 _ _]
            tunnel: [_ w427 _ w471] -> w422
            tunnel: w421 -> [_ _ w468 _]
            tunnel: [_ _ w467 _] -> _
            tunnel: w419 -> [_ w426 w466 _]
            event "stop": Value Change {
              n113 = event-data() -> ()  [unwired: 1 in, 6 out]
              n114 = local read "stop"() -> (w425:bool)
            }
            event Value Change {
              # "Live video for Calibration and 2D\nScan Modes.\n\nIdle Video for MultiD Scan modes\nUNTIL Begin Scan Button pressed?\n\nMultiD is waiting for trigger"
              n115 = event-data() -> ("NewVal"=w429:T1)  [unwired: 1 in, 5 out]
              n116 = Unbundle By Name(w429) -> ("Mode"=w428:enum16{"X", "XY", "XYZ", "XYZT", "XYZC"})
              n117 = case shown="\"XYZ\"" w428 {
                tunnel: w430 -> [w441 w453 w462 _ _]
                tunnel: w429 -> [w433 w445 w456 w464 w465]
                tunnel: [w433 w445 w456 w464 w465] -> w427
                tunnel: w426 -> [w432 w444 _ _ _]
                frame "X" {
                  w435 = ModeEnum."generateWaves"  # Mode
                  w436 = 0 ("timeout in ms (-1)")
                  w431 = 1.0 items=["Internal"=1.0, "External"=2.0] ("Trigger Source")
                  n118 = property on="Trigger Source" class="Ring (strict)"("Value"=w431) -> ()  [unwired: 2 in, 2 out]
                  n119 = Bundle("Enum"=CameraControlTypeDef."Readout Mode", "Trigger Source"=w431, "timeout in ms (-1)"=w436) -> (w440:T15)  [unwired: 1 in]
                  n120 = Enqueue Element(queue=w441, element=w440) -> (queue out=w438:refnum<queue>)  [unwired: 2 in, 2 out]
                  n121 = Bundle("Enum"=CameraControlTypeDef."Preview", "Trigger Source"=w431, "timeout in ms (-1)"=w436) -> (w439:T15)  [unwired: 1 in]
                  n122 = Bundle("Mode"=w435, "NewVal"=w433) -> (w434:cluster{"Mode":T7, "NewVal":T1})  [unwired: 1 in]
                  n123 = Enqueue Element(queue=w438, element=w439) -> ()  [unwired: 2 in, 3 out]
                  n124 = Enqueue Element(queue=w432, element=w434) -> ()  [unwired: 2 in, 3 out]
                }
                frame "XY" {
                  w447 = ModeEnum."generateWaves"  # Mode
                  w448 = 0 ("timeout in ms (-1)")
                  w443 = 2.0 items=["Internal"=1.0, "External"=2.0] ("Trigger Source")
                  n125 = property on="Trigger Source" class="Ring (strict)"("Value"=w443) -> ()  [unwired: 2 in, 2 out]
                  n126 = Bundle("Enum"=CameraControlTypeDef."Readout Mode", "Trigger Source"=w443, "timeout in ms (-1)"=w448) -> (w452:T15)  [unwired: 1 in]
                  n127 = Enqueue Element(queue=w453, element=w452) -> (queue out=w449:refnum<queue>)  [unwired: 2 in, 2 out]
                  n128 = Bundle("Mode"=w447, "NewVal"=w445) -> (w446:cluster{"Mode":T7, "NewVal":T1})  [unwired: 1 in]
                  n129 = Bundle("Enum"=CameraControlTypeDef."Preview", "Trigger Source"=w443, "timeout in ms (-1)"=w448) -> (w451:T15)  [unwired: 1 in]
                  n130 = Enqueue Element(queue=w444, element=w446) -> ()  [unwired: 2 in, 3 out]
                  n131 = Enqueue Element(queue=w449, element=w451) -> ()  [unwired: 2 in, 3 out]
                  n132 = property on="Microscope Settings" class="Clust (strict)" props=["Value"]() -> ()  [unwired: 2 in, 3 out]
                }
                frame "XYZ" {
                  w457 = 0 ("timeout in ms (-1)")
                  w455 = 2.0 items=["Internal"=1.0, "External"=2.0] ("Trigger Source")
                  n133 = property on="Trigger Source" class="Ring (strict)"("Value"=w455) -> ()  [unwired: 2 in, 2 out]
                  n134 = Bundle("Enum"=CameraControlTypeDef."Readout Mode", "Trigger Source"=w455, "timeout in ms (-1)"=w457) -> (w461:T15)  [unwired: 1 in]
                  n135 = Enqueue Element(queue=w462, element=w461) -> (queue out=w460:refnum<queue>)  [unwired: 2 in, 2 out]
                  n136 = Bundle("Enum"=CameraControlTypeDef."Idle", "Trigger Source"=w455, "timeout in ms (-1)"=w457) -> (w459:T15)  [unwired: 1 in]
                  n137 = Enqueue Element(queue=w460, element=w459) -> ()  [unwired: 2 in, 3 out]
                }
                frame "XYZT" {
                }
                frame "XYZC" {
                }
              }
            }
            event "Scan": Value Change {
              w470 = ModeEnum."runWaves"  # Mode
              n138 = event-data() -> ()  [unwired: 1 in, 6 out]
              n139 = Bundle("Mode"=w470, "Value"=w468) -> (w469:cluster{"Mode":T7, "Value":T1})  [unwired: 1 in]
              n140 = Enqueue Element(queue=w466, element=w469) -> (queue out=w467:refnum<queue>)  [unwired: 2 in, 2 out]
            }
            event Timeout {
              n141 = event-data() -> ()  [unwired: 1 in, 3 out]
              n142 = property on="Microscope Settings" class="Clust (strict)"() -> ("Value"=w471:T1)  [unwired: 2 in, 2 out]
            }
          }
        }
        n143 = Merge Errors(w177, w178) -> (w179:errorcluster)
      }
      frame "deinit" {
        n144 = call <vilib>:"DAQmx Stop Task.vi"("task/channels in"=w482) -> ("task out"=w483:refnum<k21>)  [unwired: 13 in, 1 out]
        n145 = call <vilib>:"DAQmx Stop Task.vi"("task/channels in"=w484) -> ("task out"=w485:refnum<k21>)  [unwired: 13 in, 1 out]
        n146 = call <vilib>:"DAQmx Clear Task.vi"("task in"=w483) -> ("error out"=w479:errorcluster)  [unwired: 14 in]
        n147 = call "tm_stopcapture.vi"("error in (no error)"=w494, "Handle in"=w490) -> ("error out"=w497:errorcluster, "Handle out"=w496:u32)  [unwired: 8 in]
        n148 = call <vilib>:"DAQmx Clear Task.vi"("task in"=w485) -> ("error out"=w480:errorcluster)  [unwired: 14 in]
        n149 = call "tm_unpreparecapture.vi"("error in (no error)"=w497, "Handle in"=w496) -> ("error out"=w498:errorcluster, "Handle out"=w495:u32)  [unwired: 8 in]
        n150 = call "tm_closecamera.vi"("error in (no error)"=w498, "Handle in"=w495) -> ("error out"=w499:errorcluster)  [unwired: 9 in]
        n151 = Flush Queue(queue=w472) -> (queue out=w478:refnum<queue>)  [unwired: 1 in, 2 out]
        n152 = call "tm_deinitialize.vi"("error in (no error)"=w499) -> ("error out"=w475:errorcluster)  [unwired: 10 in]
        n153 = Release Queue(queue=w473, error in (no error)=w475) -> (error out=w492:errorcluster)  [unwired: 1 in, 2 out]
        n154 = Release Queue(queue=w478) -> (error out=w481:errorcluster)  [unwired: 2 in, 2 out]
        n155 = Flush Queue(queue=w477, error in (no error)=w475) -> (queue out=w476:refnum<queue>, error out=w474:errorcluster)  [unwired: 1 out]
        n156 = Release Queue(queue=w476, error in (no error)=w474) -> (error out=w491:errorcluster)  [unwired: 1 in, 2 out]
        n157 = Merge Errors(w492, w491, w481, w480, w479) -> (w493:errorcluster)
      }
    }
    n158 = Or(x="stop", y=w16) -> (x .or. y?=w17:bool)
  }
  "error IO" <- w4
  n159 = disable-structure shown="Enabled" {
    frame Disabled {
      # "Parallise decode buffer"
      n160 = call "tm_startcapture_b.vi"() -> ()  [unwired: 10 in, 2 out]
      n161 = call "tm_waitnextframe.vi"() -> ()  [unwired: 8 in, 4 out]
      n162 = call "tm_getframe_a.vi"() -> ()  [unwired: 7 in, 5 out]
    }
    frame Enabled {
    }
  }
